vi "test3-SyncMessage_API.vi"(8 "error in (no error)":errorcluster, 11 "TestCase in":refnum<class "testcase-CSMMessage.lvclass">) -> (0 "error out":errorcluster, 3 "TestCase out":refnum<class "testcase-CSMMessage.lvclass">)   [LabVIEW 2017, in "testcase-CSMMessage.lvclass"]
uses:
  testcase-CSMMessage.lvclass
  31aab9b4-27f2-4601-9b9c-9d12425ab602.vi
  src/user.lib/_NEVSTOP/Communicable State Machine(CSM)/AdvanceAPI/CSM - Make String Arguments Safe.vi
  src/user.lib/_NEVSTOP/Communicable State Machine(CSM)/AdvanceAPI/CSM - Keywords.vi
  <vilib>/addons/_JKI Toolkits/VI Tester/TestCase.llb/TestCase.lvclass
  src/user.lib/_NEVSTOP/Communicable State Machine(CSM)/Communicable State Machine.lvlib
  CSM/CSM-Testcase.lvlib
  C:/Program Files (x86)/National Instruments/LabVIEW 2017/vi.lib/addons/_JKI Toolkits/VI Tester/TestCase.llb/TestCase.lvclass
panel:
  out "Loopcount":i32
  out "debug message":string
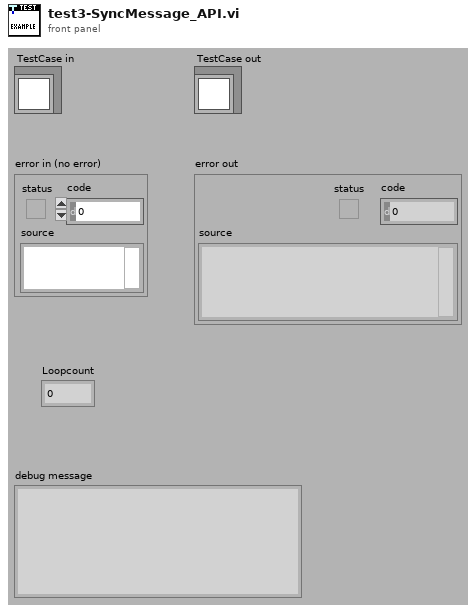
[diagram p1: front panel]
types:
  T1 = cluster{"Arguments":string, "Response":string, "error":errorcluster}
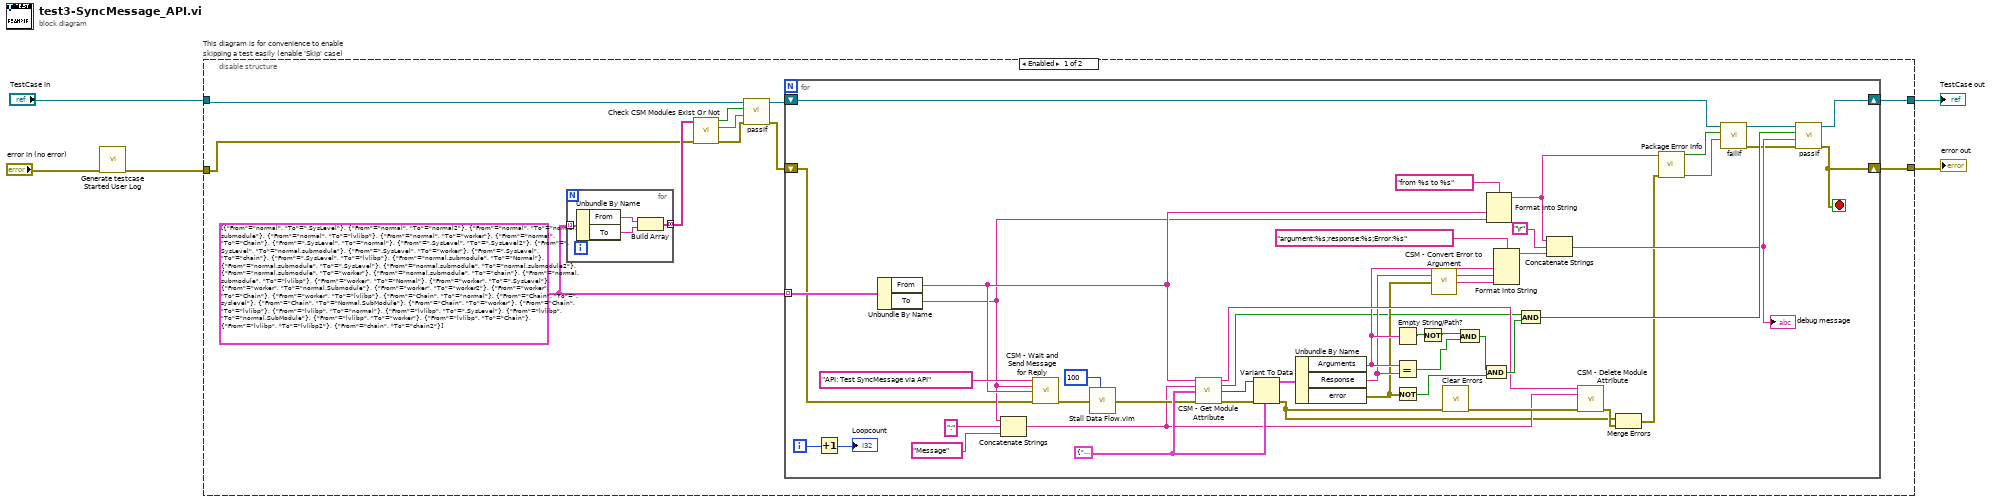
[diagram p0: block diagram]
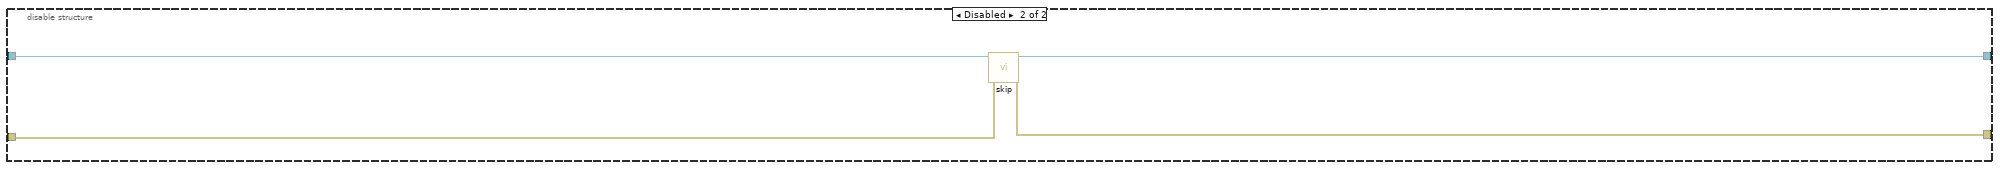
[diagram p2: hidden frame]
diagram:
  n1 = call "Generate testcase Started User Log.vi"("Error In"="error in (no error)") -> ("error out"=w1:errorcluster)  [unwired: 10 in]
  n2 = disable-structure "This diagram is for convenience to enable skipping a test easily (enable 'Skip' case)" shown="Enabled" {
    disable-tunnel: "TestCase in" -> [w9 w71]
    disable-tunnel: [w7 w69] -> w2
    disable-tunnel: [w6 w70] -> w4
    disable-tunnel: w1 -> [w10 w68]
    frame Enabled {
      w12 = cluster{"From":string, "To":string}[] [{"From"="normal", "To"=".SysLevel"}, {"From"="normal", "To"="normal2"}, {"From"="normal", "To"="normal.submodule"}, {"From"="normal", "To"="lvlibp"}, {"From"="normal", "To"="worker"}, {"From"="normal", "To"="Chain"}, {"From"=".SysLevel", "To"="normal"}, {"From"=".SysLevel", "To"=".SysLevel2"}, {"From"=".SysLevel", "To"="normal.submodule"}, {"From"=".SysLevel", "To"="worker"}, {"From"=".SysLevel", "To"="chain"}, {"From"=".SysLevel", "To"="lvlibp"}, {"From"="normal.submodule", "To"="Normal"}, {"From"="normal.submodule", "To"=".SysLevel"}, {"From"="normal.submodule", "To"="normal.submodule2"}, {"From"="normal.submodule", "To"="worker"}, {"From"="normal.submodule", "To"="chain"}, {"From"="normal.submodule", "To"="lvlibp"}, {"From"="worker", "To"="Normal"}, {"From"="worker", "To"=".SysLevel"}, {"From"="worker", "To"="normal.Submodule"}, {"From"="worker", "To"="worker2"}, {"From"="worker", "To"="Chain"}, {"From"="worker", "To"="lvlibp"}, {"From"="Chain", "To"="normal"}, {"From"="Chain", "To"=".syslevel"}, {"From"="Chain", "To"="Normal.SubModule"}, {"From"="Chain", "To"="worker"}, {"From"="Chain", "To"="lvlibp"}, {"From"="lvlibp", "To"="normal"}, {"From"="lvlibp", "To"=".SysLevel"}, {"From"="lvlibp", "To"="normal.SubModule"}, {"From"="lvlibp", "To"="worker"}, {"From"="lvlibp", "To"="Chain"}, {"From"="lvlibp", "To"="lvlibp2"}, {"From"="chain", "To"="chain2"}]
      n3 = for {
        tunnel: w12 -> [w20] mode=indexing
        tunnel: [w17] -> w15 mode=concatenating
        n4 = Unbundle By Name(w20) -> ("From"=w19:string, "To"=w18:string)
        n5 = Build Array(w19, w18) -> (w17:string[])
      }
      n6 = call "Check CSM Modules Exist Or Not.vi"("error in"=w10, "CSM names in"=w15) -> ("error out"=w13:errorcluster, "Debug string"=w14:string, "All Modules Exist?"=w16:bool)  [unwired: 7 in]
      n7 = call-dynamic "passIf.vi"("error in (no error)"=w13, "message (\"\")"=w14, "pass"=w16, "TestCase in"=w9) -> ("error out"=w11:errorcluster, "TestCase out"=w8:refnum<class "testcase-CSMMessage.lvclass">)  [unwired: 6 in]
      n8 = for {
        tunnel: w12 -> [w60] mode=indexing
        shift-right: [w67] -> w7
        shift-left: w8 -> [w23]
        shift-right: [w43] -> w6
        shift-left: w11 -> [w30]
        i -> [w36]
        stop <- w43 stop-if-true
        w64 = T1 {"Arguments"="", "Response"="", "error"={"status"=FALSE, "code"=0, "source"=""}}
        n9 = Increment(x=w36) -> (x+1=→"Loopcount":i32)
        n10 = Unbundle By Name(w60) -> ("From"=w40:string, "To"=w38:string)
        n11 = Concatenate Strings(w38, ":" ("string"), "Message" ("string")) -> (w39:string)
        n12 = call "CSM - Wait and Send Message for Reply.vi"("State"="API: Test SyncMessage via API", "Arguments (\"\")"=w38, "Target Module"=w40, "Error In (No Error)"=w30) -> ("error out"=w32:errorcluster)  [unwired: 8 in, 3 out]
        n13 = call "Stall Data Flow.vim"("value in"=w32, "milliseconds to wait"=u32 100) -> ("value out"=w47:errorcluster)  [unwired: 1 out]
        n14 = call "CSM - Get Module Attribute.vi"("CSM Name"=w40, "Attribute"=w39, "Default Value (Empty Variant)"=w64, "Error In"=w47) -> ("CSM Name (Dup)"=w58:string, "Found"=w34:bool, "Value"=w37:variant, "error out"=w65:errorcluster)  [unwired: 7 in, 1 out]
        n15 = Variant To Data(error in=w65, type=w64, Variant=w37) -> (data=w33:T1, error out=w28:errorcluster)
        n16 = Unbundle By Name(w33) -> ("Arguments"=w53:string, "Response"=w52:string, "error"=w50:errorcluster)
        n17 = Empty String/Path?(string/path=w53) -> (empty?=w57:bool)
        n18 = Equal?(x=w53, y=w52) -> (x = y?=w55:bool)
        n19 = Not(x=w50) -> (.not. x?=w63:bool)
        n20 = Not(x=w57) -> (.not. x?=w56:bool)
        n21 = call "CSM - Convert Error to Argument.vi"("Error"=w50) -> ("Argument"=w51:string)  [unwired: 4 in]
        n22 = call <vilib>:"Clear Errors.vi"("error in (no error)"=w28) -> ("error out"=w44:errorcluster)  [unwired: 5 in, 1 out]
        n23 = And(x=w56, y=w55) -> (x .and. y?=w54:bool)
        n24 = And(x=w54, y=w63) -> (x .and. y?=w62:bool)
        n25 = Format Into String(format string="from %s to %s", w40, w38) -> (resulting string=w24:string)  [unwired: 2 in, 1 out]
        n26 = Format Into String(format string="argument:%s;response:%s;Error:%s", w53, w52, w51) -> (resulting string=w49:string)  [unwired: 2 in, 1 out]
        n27 = And(x=w34, y=w62) -> (x .and. y?=w61:bool)
        n28 = Concatenate Strings(w24, "\r", w49) -> (w46:string)
        "debug message" <- w46
        n29 = call "CSM - Delete Module Attribute.vi"("CSM Name"=w58, "Attribute"=w39, "Error In"=w44) -> ("error out"=w29:errorcluster)  [unwired: 9 in, 3 out]
        n30 = Merge Errors(w28, w29) -> (w25:errorcluster)
        n31 = call "Package Error Info.vi"("error in"=w25, "String in"=w24) -> ("packed error info out"=w27:string, "error status"=w26:bool)  [unwired: 8 in]
        n32 = call-dynamic "failIf.vi"("message (\"\")"=w27, "fail"=w26, "TestCase in"=w23) -> ("error out"=w21:errorcluster, "TestCase out"=w22:refnum<class "testcase-CSMMessage.lvclass">)  [unwired: 7 in]
        n33 = call-dynamic "passIf.vi"("error in (no error)"=w21, "message (\"\")"=w46, "pass"=w61, "TestCase in"=w22) -> ("error out"=w43:errorcluster, "TestCase out"=w67:refnum<class "testcase-CSMMessage.lvclass">)  [unwired: 6 in]
      }
    }
    frame Disabled {
      # "skip test result while test is under development"
      n34 = call <vilib>:"skip.vi"("error in (no error)"=w68, "TestCase in"=w71) -> ("error out"=w70:errorcluster, "TestCase out"=w69:refnum<class "testcase-CSMMessage.lvclass">)  [unwired: 8 in]
    }
  }
  "error out" <- w4
  "TestCase out" <- w2
